vi "Get State.vi"(6 "Controller name":string, 8 "error in (no error)":errorcluster, 11 "Stepper in":refnum<class "Stepper.lvclass">) -> (0 "error out":errorcluster, 1 "Result ready":bool, 2 "Armed":bool, 3 "Stepper out":refnum<class "Stepper.lvclass">, 4 "Check again":bool)   [LabVIEW 2021, in "Stepper.lvclass"]
uses:
  Stepper.lvclass
  Continuous Recorder Actor/Continuous Recorder Actor.lvclass
  Measurements/Response Synchronizer/Response Synchronizer.lvclass
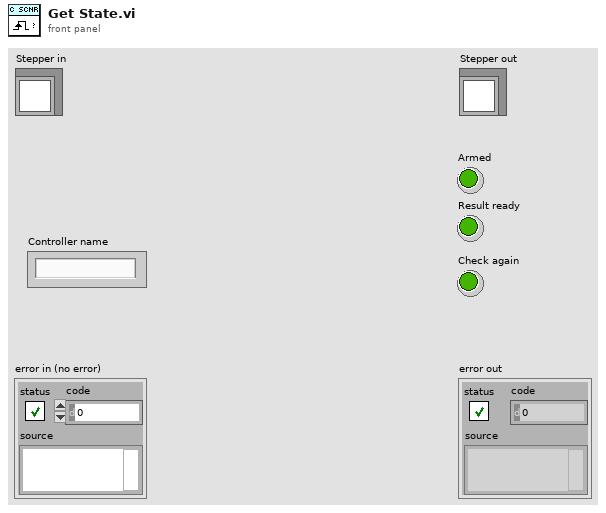
[diagram p1: front panel]
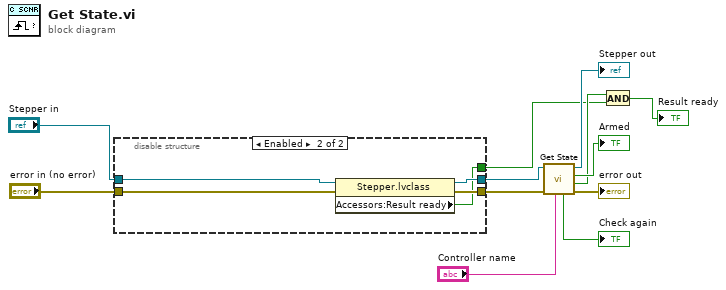
[diagram p0: block diagram]
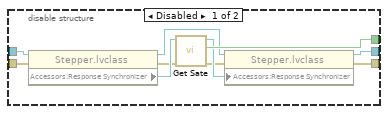
[diagram p2: hidden frame]
diagram:
  n1 = disable-structure shown="Enabled" {
    disable-tunnel: "error in (no error)" -> [w22 w27]
    disable-tunnel: "Stepper in" -> [w21 w26]
    disable-tunnel: [w18 w23] -> w3
    disable-tunnel: [w14 w24] -> w2
    disable-tunnel: [w13 w25] -> w1
    frame Disabled {
      n2 = property class="Stepper.lvclass"(reference=w21, error in=w22) -> (reference out=w15:refnum<class "Stepper.lvclass">, error out=w19:errorcluster, "Accessors:Response Synchronizer"=w20:refnum<class "Response Synchronizer.lvclass">)
      n3 = call-dynamic "Get Sate.vi"("error in (no error)"=w19, "Response Synchronizer in"=w20) -> ("error out"=w16:errorcluster, "Result ready"=w18:bool, "Response Synchronizer out"=w17:refnum<class "Response Synchronizer.lvclass">)  [unwired: 6 in, 1 out]
      n4 = property class="Stepper.lvclass"(reference=w15, error in=w16, "Accessors:Response Synchronizer"=w17) -> (reference out=w14:refnum<class "Stepper.lvclass">, error out=w13:errorcluster)
    }
    frame Enabled {
      n5 = property class="Stepper.lvclass"(reference=w26, error in=w27) -> (reference out=w24:refnum<class "Stepper.lvclass">, error out=w25:errorcluster, "Accessors:Result ready"=w23:bool)
    }
  }
  n6 = call-parent "Get State.vi"("Controller name"="Controller name", "error in (no error)"=w1, "Instrument Actor in"=w2) -> ("error out"=→"error out":errorcluster, "Result ready"=w5:bool, "Armed"=→"Armed":bool, "Instrument Actor out"=→"Stepper out":refnum<class "Stepper.lvclass">, "Check again"=→"Check again":bool)  [unwired: 4 in]
  n7 = And(x=w5, y=w3) -> (x .and. y?=→"Result ready":bool)
